vi "MasterBatch.vi"(0 "Drop Time":i32, 1 "Cloud center":i32[](array[numeric]), 2 "ROI Radius":i32, 3 "Window Radius":i32, 4 "Base Filename":string, 5 "Master Batch File":path, 7 "Write Batch?":bool) -> ()   [LabVIEW 2013]
doc: "Write Master Batch File of scan parameters based on File Patch and scan variables"
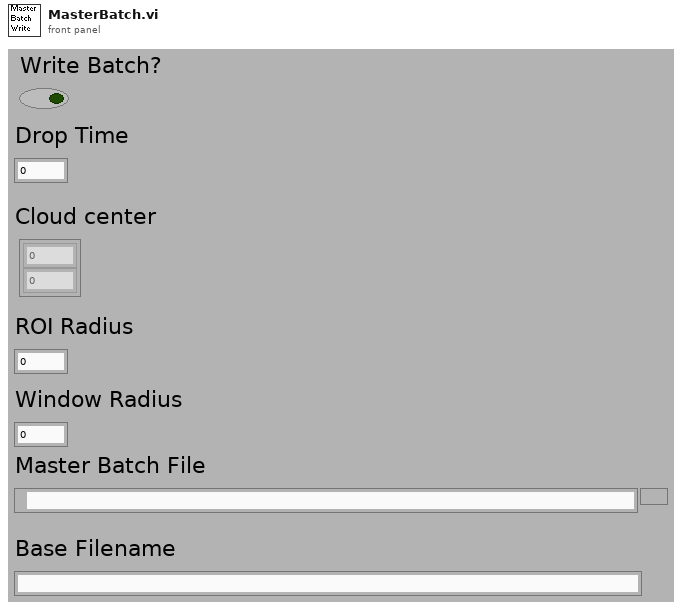
[diagram p1: front panel]
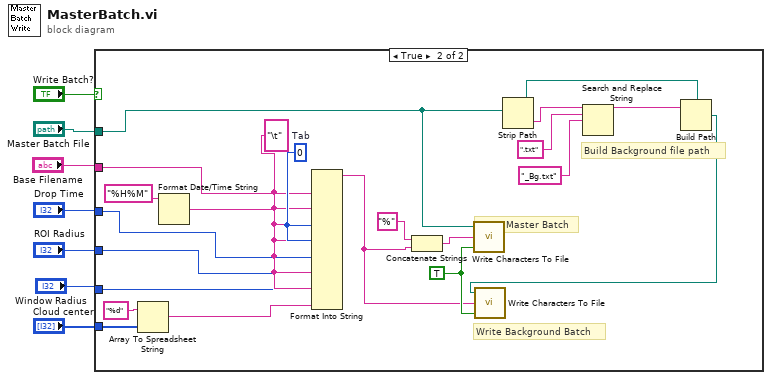
[diagram p0: block diagram]
diagram:
  n1 = case shown="True" "Write Batch?" {
    tunnel: "Base Filename" -> [_ w25]
    tunnel: "Master Batch File" -> [_ w23]
    tunnel: "Drop Time" -> [_ w26]
    tunnel: "ROI Radius" -> [_ w10]
    tunnel: "Cloud center" -> [_ w28]
    tunnel: "Window Radius" -> [_ w9]
    frame False {
    }
    frame True {
      w17 = TRUE ("append to file? (new file:F)")
      w27 = 0
      w24 = "\t"  # Tab
      # "Write Background Batch"
      # "Write Master Batch"
      # "Build Background file path"
      n2 = Array To Spreadsheet String(array=w28, 3:"%d" ("format string")) -> (spreadsheet string=w8:string)  [unwired: 1 in]
      n3 = Format Date/Time String(time format string (%c)="%H%M") -> (date/time string=w14:string)  [unwired: 2 in]
      n4 = Format Into String(w25, w24, w14, w24, w27, w24, w27, w24, w26, w24, w10, w24, w9, w24, w8) -> (resulting string=w11:string)  [unwired: 3 in, 1 out]
      n5 = Concatenate Strings("%", w11) -> (w13:string)
      n6 = call <vilib>:"Write Characters To File.vi"("append to file? (new file:F)"=w17, "character string"=w13, "file path (dialog if empty)"=w23) -> ()  [unwired: 2 in, 1 out]
      n7 = Strip Path(path=w23) -> (stripped path=w19:path, name=w22:string)
      n8 = Search and Replace String(input string=w22, search string=".txt", replace string="_Bg.txt") -> (result string=w18:string)  [unwired: 5 in, 3 out]
      n9 = Build Path(base path=w19, name or relative path=w18) -> (appended path=w16:path)
      n10 = call <vilib>:"Write Characters To File.vi"("append to file? (new file:F)"=w17, "character string"=w11, "file path (dialog if empty)"=w16) -> ()  [unwired: 2 in, 1 out]
    }
  }
